vi "Validate Limits.vi"(10 "Limits":cluster{"Upper Limit":u8, "Lower Limit":u8}) -> (2 "valid?":bool, 3 "Limits out":cluster{"Upper Limit":u8, "Lower Limit":u8})   [LabVIEW 2020, in "Digital Acquisition.lvlib" / "Digital Acquisition.lvclass"]
uses:
  Digital Acquisition/Digital Acquisition.lvclass
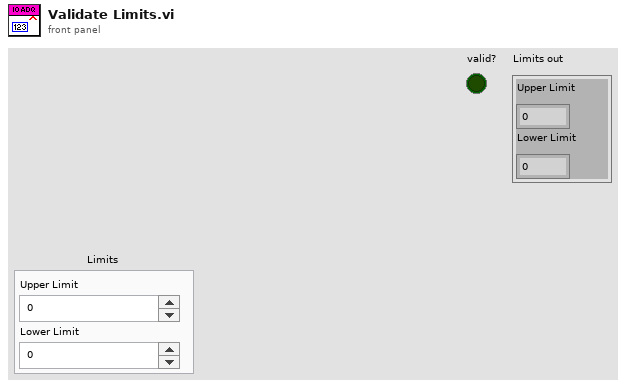
[diagram p1: front panel]
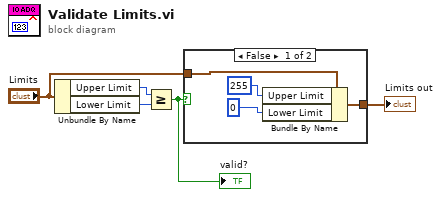
[diagram p0: block diagram]
diagram:
  n1 = Unbundle By Name("Limits") -> ("Upper Limit"=w5:u8, "Lower Limit"=w4:u8)
  n2 = Greater Or Equal?(x=w5, y=w4) -> (x >= y?=w3:bool)
  "valid?" <- w3
  n3 = case shown="False" w3 {
    tunnel: "Limits" -> [w9 w10]
    tunnel: [w8 w10] -> w1
    frame False {
      n4 = Bundle By Name(cluster=w9, "Upper Limit"=u8 255, "Lower Limit"=u8 0) -> (w8:cluster{"Upper Limit":u8, "Lower Limit":u8})
    }
    frame True {
    }
  }
  "Limits out" <- w1
